vi "VisaBasicForScan.vi"(1 "VISA resource name":refnum<visa-resource-name>, 2 "Cmd":string, 3 "TimeOut":bool=TRUE, 4 "Time(0.1)":u32=10, 5 "error in (no error)":errorcluster, 8 "VisaAction":enum16{"Open", "Send", "Recieve", "Close"}(ring)) -> (16 "read string":string, 19 "error out":errorcluster)   [LabVIEW 2019]
uses:
  <vilib>/Instr/_visa.llb/VISA Configure Serial Port (Instr).vi
  LLB/Commonly VI.lvlib
panel:
  out "Numeric":i32
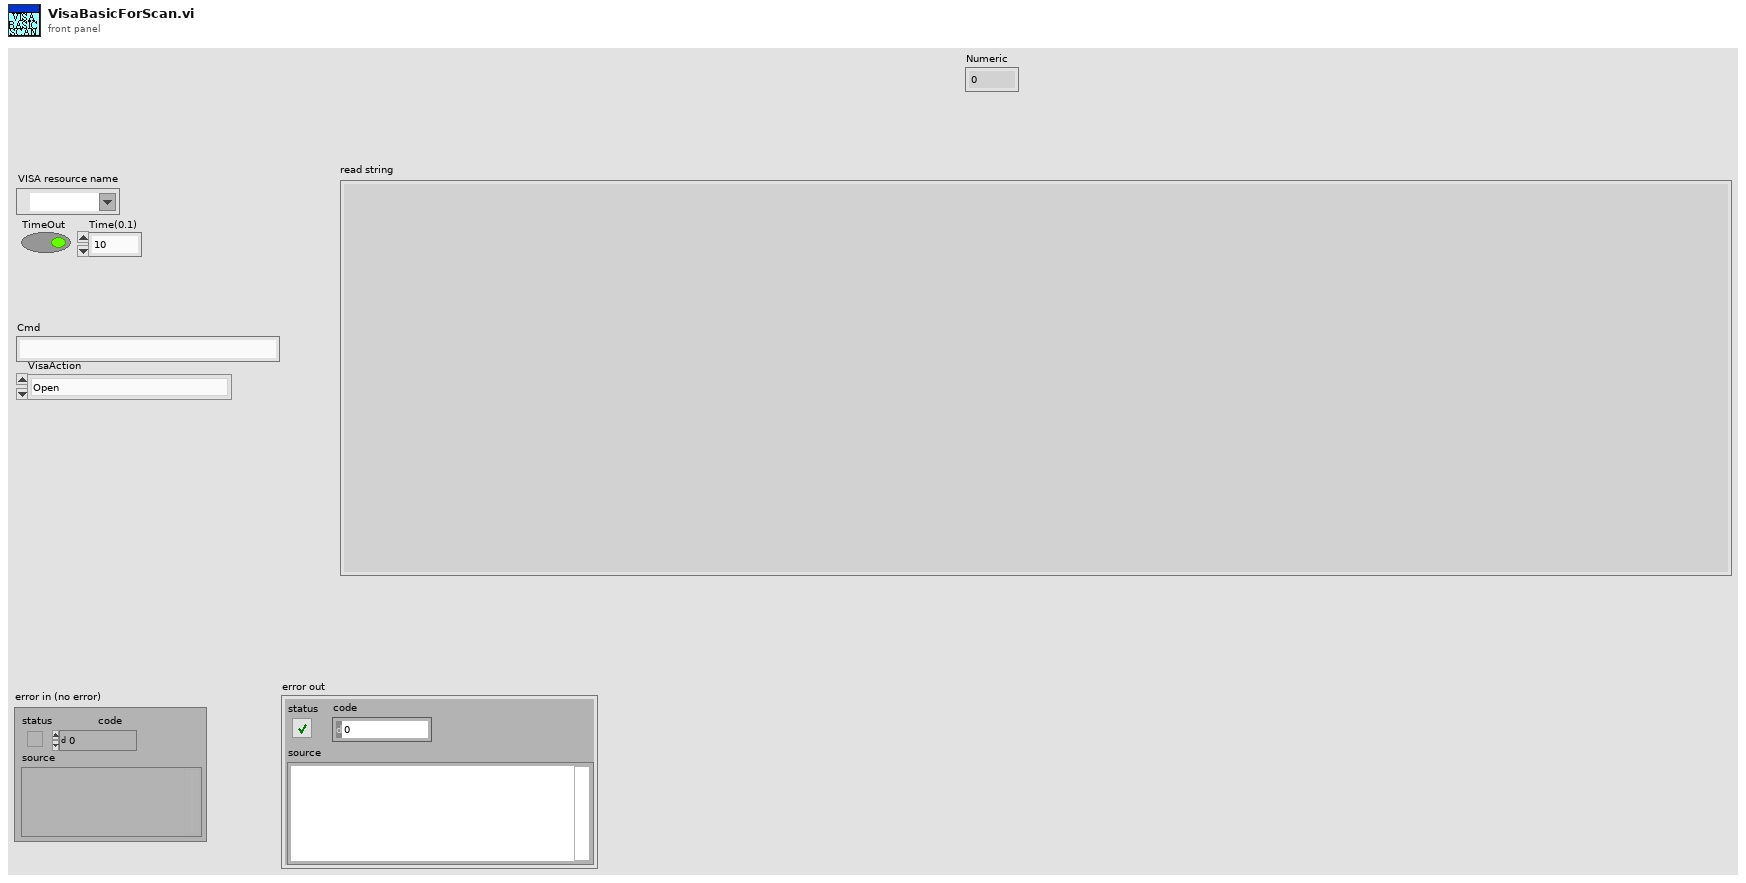
[diagram p1: front panel]
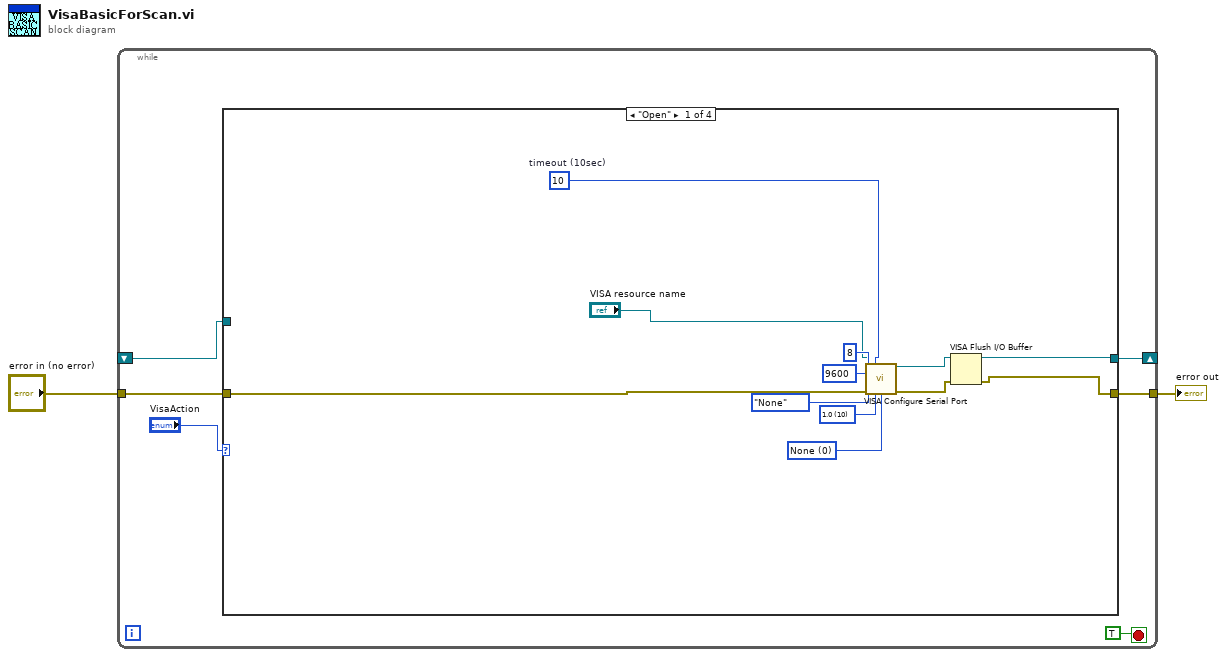
[diagram p0: block diagram]
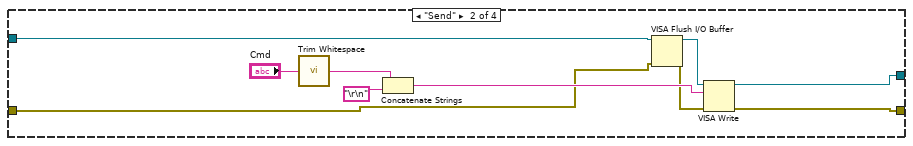
[diagram p2: hidden frame]
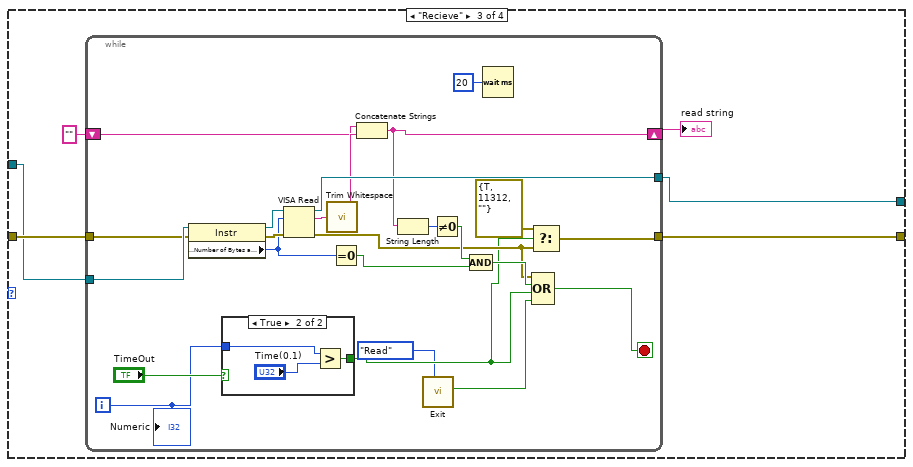
[diagram p3: hidden frame]
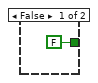
[diagram p4: hidden frame]
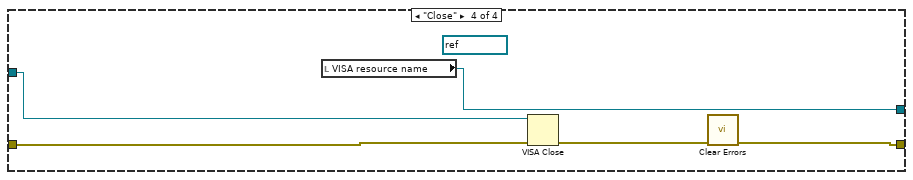
[diagram p5: hidden frame]
diagram:
  n1 = while {
    tunnel: "error in (no error)" -> [w6]
    tunnel: [w7] -> w2
    shift-right: [w4] -> _
    shift-left: _ -> [w3]
    stop <- TRUE stop-if-true
    n2 = case shown="\"Open\"" "VisaAction" {
      tunnel: [w10 w30 w35 w66] -> w7
      tunnel: w6 -> [w20 w21 w36 w68]
      tunnel: w3 -> [_ w22 w32 w67]
      tunnel: [w11 w25 w31 w65] -> w4
      frame "Open" {
        w15 = u16 0 items=["None", "XON/XOFF", "RTS/CTS", "XON/XOFF & RTS/CTS", "DTR/DSR", "XON/XOFF & DTR/DSR"] ("flow control (0:none)")
        w16 = u16 10 items=["1.0"=10, "1.5"=15, "2.0"=20] ("stop bits (10: 1 bit)")
        w19 = u32 10  # timeout (10sec)
        n3 = call-poly "VISA Configure Serial Port"("VISA resource name"="VISA resource name", "timeout (10sec)"=w19, "baud rate (9600)"=u32 9600, "data bits (8)"=u16 8, "parity (0:none)"=enum16{"None", "Odd", "Even", "Mark", "Space"}."None", "error in (no error)"=w20, "stop bits (10: 1 bit)"=w16, "flow control (0:none)"=w15) -> ("VISA resource name out"=w12:refnum<visa-resource-name>, "error out"=w9:errorcluster)  [unwired: 1 in, 5 out]
        n4 = VISA Flush I/O Buffer(VISA resource name=w12, error in (no error)=w9) -> (VISA resource name out=w11:refnum<visa-resource-name>, error out=w10:errorcluster)  [unwired: 1 in]
      }
      frame "Send" {
        n5 = call <vilib>:"Trim Whitespace.vi"("string"="Cmd") -> ("trimmed string"=w26:string)  [unwired: 1 in]
        n6 = Concatenate Strings(w26, "\r\n") -> (w27:string)
        n7 = VISA Flush I/O Buffer(VISA resource name=w22, error in (no error)=w21) -> (VISA resource name out=w23:refnum<visa-resource-name>, error out=w24:errorcluster)  [unwired: 1 in]
        n8 = VISA Write(VISA resource name=w23, write buffer=w27, error in (no error)=w24) -> (VISA resource name out=w25:refnum<visa-resource-name>, error out=w30:errorcluster)  [unwired: 1 out]
      }
      frame "Recieve" {
        n9 = while {
          tunnel: w32 -> [w58]
          tunnel: w36 -> [w57]
          tunnel: [w56] -> w31
          tunnel: [w51] -> w35
          shift-right: [w48] -> w34
          shift-left: "" ("trimmed string") -> [w54]
          i -> [w39]
          stop <- w52 stop-if-true
          n10 = property class="Instr"(reference=w58, error in=w57) -> (reference out=w59:refnum<visa-resource-name>, error out=w60:errorcluster, "Serial Settings:Number of Bytes at Serial Port"=w40:u32)
          n11 = case shown="True" "TimeOut" {
            tunnel: w39 -> [_ w64]
            tunnel: [FALSE w62] -> w38
            frame False {
            }
            frame True {
              n12 = Greater?(x=w64, y="Time(0.1)") -> (0:w62:bool)
            }
          }
          n13 = VISA Read(VISA resource name=w59, byte count=w40, error in (no error)=w60) -> (VISA resource name out=w56:refnum<visa-resource-name>, read buffer=w42:string, error out=w44:errorcluster)  [unwired: 1 out]
          n14 = call <vilib>:"Trim Whitespace.vi"("string"=w42) -> ("trimmed string"=w55:string)  [unwired: 1 in]
          n15 = Equal To 0?(x=w40) -> (x = 0?=w49:bool)
          n16 = Concatenate Strings(w54, w55) -> (w48:string)
          n17 = String Length(string=w48) -> (length=w47:i32)
          n18 = call "Exit.vi"("Enum"=enum16{"Initial", "Read", "Write"}."Read") -> ("ExitOut"=w43:bool)  [unwired: 10 in]
          n19 = Not Equal To 0?(x=w47) -> (x != 0?=w46:bool)
          n20 = Compound Arithmetic op=AND(w46, w49) -> (w45:bool)
          n21 = Wait (ms)(milliseconds to wait=u32 20) -> ()  [unwired: 1 out]
          n22 = Select(t=errorcluster {"status"=TRUE, "code"=11312, "source"=""}, s=w38, f=w44) -> (s? t:f=w51:errorcluster)
          n23 = Compound Arithmetic op=OR(w44, w45, w38, w43) -> (w52:bool)
          "Numeric" <- w39
        }
        "read string" <- w34
      }
      frame "Close" {
        (unwired) refnum<visa-resource-name> "COM3" ("VISA resource name out")
        n24 = local read "VISA resource name"() -> (w65:refnum<visa-resource-name>)
        n25 = VISA Close(VISA resource name=w67, error in (no error)=w68) -> (error out=w69:errorcluster)
        n26 = call <vilib>:"Clear Errors.vi"("error in (no error)"=w69) -> ("error out"=w66:errorcluster)  [unwired: 5 in, 1 out]
      }
    }
  }
  "error out" <- w2
